vi "6733_88_write_waveform_2014.11.21.vi"(8 "Error In":errorcluster, 9 "Control Reference \nCluster Input":T1, 11 "Red MOT 88 Inputs":T2={"Active Device"="6733_Red_88", "Active Channels"=[TRUE, FALSE, FALSE, FALSE, FALSE, FALSE, FALSE, FALSE], "Waveform Parameters"=[[{"Function"=enum."Polynomial", "Initial"=0.0, "Final"=1.0, "Degree"=1.0, "Nickname"="", "Conversion"=enum."B Field Grad (G/cm)", "Constant"=0.0}, {"Function"=enum."Exponential", "Initial"=0.0, "Final"=0.0, "Degree"=1.0, "Nickname"="", "Conversion"=enum."B Field Grad (G/cm)", "Constant"=0.0}, {"Function"=enum."Exponential", "Initial"=0.0, "Final"=0.0, "Degree"=1.0, "Nickname"="", "Conversion"=enum."B Field Grad (G/cm)", "Constant"=0.0}, {"Function"=enum."Exponential", "Initial"=0.0, "Final"=0.0, "Degree"=1.0, "Nickname"="", "Conversion"=enum."B Field Grad (G/cm)", "Constant"=0.0}, {"Function"=enum."Exponential", "Initial"=0.0, "Final"=0.0, "Degree"=1.0, "Nickname"="", "Conversion"=enum."B Field Grad (G/cm)", "Constant"=0.0}, {"Function"=enum."Exponential", "Initial"=0.0, "Final"=0.0, "Degree"=1.0, "Nickname"="", "Conversion"=enum."B Field Grad (G/cm)", "Constant"=0.0}], [{"Function"=enum."Exponential", "Initial"=0.0, "Final"=0.0, "Degree"=1.0, "Nickname"="", "Conversion"=enum."B Field Grad (G/cm)", "Constant"=0.0}, {"Function"=enum."Exponential", "Initial"=0.0, "Final"=0.0, "Degree"=1.0, "Nickname"="", "Conversion"=enum."B Field Grad (G/cm)", "Constant"=0.0}, {"Function"=enum."Exponential", "Initial"=0.0, "Final"=0.0, "Degree"=1.0, "Nickname"="", "Conversion"=enum."B Field Grad (G/cm)", "Constant"=0.0}, {"Function"=enum."Exponential", "Initial"=0.0, "Final"=0.0, "Degree"=1.0, "Nickname"="", "Conversion"=enum."B Field Grad (G/cm)", "Constant"=0.0}, {"Function"=enum."Exponential", "Initial"=0.0, "Final"=0.0, "Degree"=1.0, "Nickname"="", "Conversion"=enum."B Field Grad (G/cm)", "Constant"=0.0}, {"Function"=enum."Exponential", "Initial"=0.0, "Final"=0.0, "Degree"=1.0, "Nickname"="", "Conversion"=enum."B Field Grad (G/cm)", "Constant"=0.0}], [{"Function"=enum."Exponential", "Initial"=0.0, "Final"=0.0, "Degree"=1.0, "Nickname"="", "Conversion"=enum."B Field Grad (G/cm)", "Constant"=0.0}, {"Function"=enum."Exponential", "Initial"=0.0, "Final"=0.0, "Degree"=1.0, "Nickname"="", "Conversion"=enum."B Field Grad (G/cm)", "Constant"=0.0}, {"Function"=enum."Exponential", "Initial"=0.0, "Final"=0.0, "Degree"=1.0, "Nickname"="", "Conversion"=enum."B Field Grad (G/cm)", "Constant"=0.0}, {"Function"=enum."Exponential", "Initial"=0.0, "Final"=0.0, "Degree"=1.0, "Nickname"="", "Conversion"=enum."B Field Grad (G/cm)", "Constant"=0.0}, {"Function"=enum."Exponential", "Initial"=0.0, "Final"=0.0, "Degree"=1.0, "Nickname"="", "Conversion"=enum."B Field Grad (G/cm)", "Constant"=0.0}, {"Function"=enum."Exponential", "Initial"=0.0, "Final"=0.0, "Degree"=1.0, "Nickname"="", "Conversion"=enum."B Field Grad (G/cm)", "Constant"=0.0}], [{"Function"=enum."Exponential", "Initial"=0.0, "Final"=0.0, "Degree"=1.0, "Nickname"="", "Conversion"=enum."B Field Grad (G/cm)", "Constant"=0.0}, {"Function"=enum."Exponential", "Initial"=0.0, "Final"=0.0, "Degree"=1.0, "Nickname"="", "Conversion"=enum."B Field Grad (G/cm)", "Constant"=0.0}, {"Function"=enum."Exponential", "Initial"=0.0, "Final"=0.0, "Degree"=1.0, "Nickname"="", "Conversion"=enum."B Field Grad (G/cm)", "Constant"=0.0}, {"Function"=enum."Exponential", "Initial"=0.0, "Final"=0.0, "Degree"=1.0, "Nickname"="", "Conversion"=enum."B Field Grad (G/cm)", "Constant"=0.0}, {"Function"=enum."Exponential", "Initial"=0.0, "Final"=0.0, "Degree"=1.0, "Nickname"="", "Conversion"=enum."B Field Grad (G/cm)", "Constant"=0.0}, {"Function"=enum."Exponential", "Initial"=0.0, "Final"=0.0, "Degree"=1.0, "Nickname"="", "Conversion"=enum."B Field Grad (G/cm)", "Constant"=0.0}], [{"Function"=enum."Exponential", "Initial"=0.0, "Final"=0.0, "Degree"=1.0, "Nickname"="", "Conversion"=enum."B Field Grad (G/cm)", "Constant"=0.0}, {"Function"=enum."Exponential", "Initial"=0.0, "Final"=0.0, "Degree"=1.0, "Nickname"="", "Conversion"=enum."B Field Grad (G/cm)", "Constant"=0.0}, {"Function"=enum."Exponential", "Initial"=0.0, "Final"=0.0, "Degree"=1.0, "Nickname"="", "Conversion"=enum."B Field Grad (G/cm)", "Constant"=0.0}, {"Function"=enum."Exponential", "Initial"=0.0, "Final"=0.0, "Degree"=1.0, "Nickname"="", "Conversion"=enum."B Field Grad (G/cm)", "Constant"=0.0}, {"Function"=enum."Exponential", "Initial"=0.0, "Final"=0.0, "Degree"=1.0, "Nickname"="", "Conversion"=enum."B Field Grad (G/cm)", "Constant"=0.0}, {"Function"=enum."Exponential", "Initial"=0.0, "Final"=0.0, "Degree"=1.0, "Nickname"="", "Conversion"=enum."B Field Grad (G/cm)", "Constant"=0.0}], [{"Function"=enum."Exponential", "Initial"=0.0, "Final"=0.0, "Degree"=1.0, "Nickname"="", "Conversion"=enum."B Field Grad (G/cm)", "Constant"=0.0}, {"Function"=enum."Exponential", "Initial"=0.0, "Final"=0.0, "Degree"=1.0, "Nickname"="", "Conversion"=enum."B Field Grad (G/cm)", "Constant"=0.0}, {"Function"=enum."Exponential", "Initial"=0.0, "Final"=0.0, "Degree"=1.0, "Nickname"="", "Conversion"=enum."B Field Grad (G/cm)", "Constant"=0.0}, {"Function"=enum."Exponential", "Initial"=0.0, "Final"=0.0, "Degree"=1.0, "Nickname"="", "Conversion"=enum."B Field Grad (G/cm)", "Constant"=0.0}, {"Function"=enum."Exponential", "Initial"=0.0, "Final"=0.0, "Degree"=1.0, "Nickname"="", "Conversion"=enum."B Field Grad (G/cm)", "Constant"=0.0}, {"Function"=enum."Exponential", "Initial"=0.0, "Final"=0.0, "Degree"=1.0, "Nickname"="", "Conversion"=enum."B Field Grad (G/cm)", "Constant"=0.0}], [{"Function"=enum."Exponential", "Initial"=0.0, "Final"=0.0, "Degree"=1.0, "Nickname"="", "Conversion"=enum."B Field Grad (G/cm)", "Constant"=0.0}, {"Function"=enum."Exponential", "Initial"=0.0, "Final"=0.0, "Degree"=1.0, "Nickname"="", "Conversion"=enum."B Field Grad (G/cm)", "Constant"=0.0}, {"Function"=enum."Exponential", "Initial"=0.0, "Final"=0.0, "Degree"=1.0, "Nickname"="", "Conversion"=enum."B Field Grad (G/cm)", "Constant"=0.0}, {"Function"=enum."Exponential", "Initial"=0.0, "Final"=0.0, "Degree"=1.0, "Nickname"="", "Conversion"=enum."B Field Grad (G/cm)", "Constant"=0.0}, {"Function"=enum."Exponential", "Initial"=0.0, "Final"=0.0, "Degree"=1.0, "Nickname"="", "Conversion"=enum."B Field Grad (G/cm)", "Constant"=0.0}, {"Function"=enum."Exponential", "Initial"=0.0, "Final"=0.0, "Degree"=1.0, "Nickname"="", "Conversion"=enum."B Field Grad (G/cm)", "Constant"=0.0}], [{"Function"=enum."Exponential", "Initial"=0.0, "Final"=0.0, "Degree"=1.0, "Nickname"="", "Conversion"=enum."B Field Grad (G/cm)", "Constant"=0.0}, {"Function"=enum."Exponential", "Initial"=0.0, "Final"=0.0, "Degree"=1.0, "Nickname"="", "Conversion"=enum."B Field Grad (G/cm)", "Constant"=0.0}, {"Function"=enum."Exponential", "Initial"=0.0, "Final"=0.0, "Degree"=1.0, "Nickname"="", "Conversion"=enum."B Field Grad (G/cm)", "Constant"=0.0}, {"Function"=enum."Exponential", "Initial"=0.0, "Final"=0.0, "Degree"=1.0, "Nickname"="", "Conversion"=enum."B Field Grad (G/cm)", "Constant"=0.0}, {"Function"=enum."Exponential", "Initial"=0.0, "Final"=0.0, "Degree"=1.0, "Nickname"="", "Conversion"=enum."B Field Grad (G/cm)", "Constant"=0.0}, {"Function"=enum."Exponential", "Initial"=0.0, "Final"=0.0, "Degree"=1.0, "Nickname"="", "Conversion"=enum."B Field Grad (G/cm)", "Constant"=0.0}]], "Active Phases"=[TRUE, FALSE, FALSE, FALSE, FALSE, FALSE], "Phase Times"=[0.1, 0.1, 0.1], "Trigger Channel"="/6733_Red_88/PFI0"} {"Phase Times" format="%.0p"; "Waveform Parameters"."Degree" min=1.0}) -> (0 "error out":errorcluster={"status"=TRUE, "code"=-89125, "source"="6733_88_write_waveform_2014.11.21.vi<append>\n<B>Source Device: </B>6733_Red_88\n<B>Destination Device: </B>6733_Red_87\n\n<B>Task Name: </B>Red MOT 88 Wfm"}, 2 "counter task out":refnum<k21>, 3 "waveform task out":refnum<k21>="Red MOT 88 Wfm")   [LabVIEW 2016]
uses:
  6733_Red_MOT/6733_control_panel.ctl
  6733_Red_MOT/6733_waveform_parameter_array.ctl
  6733_Red_MOT/6733_waveform_item.ctl
  6733_Red_MOT/Neutral_voltage_conversion_control.ctl
  Controls/6733/Trigger_Channel_Selector.ctl
  Control 1.ctl
  <vilib>/DAQmx/write.llb/DAQmx Write (Analog 1D DBL NChan 1Samp).vi
  <vilib>/DAQmx/write.llb/DAQmx Write (Analog 1D Wfm NChan NSamp).vi
  <vilib>/DAQmx/miscellaneous.llb/DAQmx Fill In Error Info.vi
  <vilib>/Waveform/WDTOps.llb/WDT Append Waveforms DBL.vi
  <vilib>/Waveform/WDTOps.llb/WDT Scale Delta t DBL.vi
  <vilib>/DAQmx/configure/timing.llb/DAQmx Timing (Sample Clock).vi
  <vilib>/DAQmx/create/channels.llb/DAQmx Create Channel (CO-Pulse Generation-Frequency).vi
  <vilib>/DAQmx/configure/timing.llb/DAQmx Timing (Implicit).vi
  <vilib>/DAQmx/configure/trigger.llb/DAQmx Start Trigger (Digital Edge).vi
  <resource>/objmgr/daqmx.rc
panel:
  out "Total Time":dbl=0.1
  out "Sample Rate":dbl=163840.0
  out "Waveforms":waveform(dbl)[](graph)
  out "Max Sample Rate":dbl=1000000.0
  out "# Inactive Channels":i32=7
  out "# Active Channels":i16=1
  out "Inactive Channels":tag[](array[tag])=["6733_Red_87/ao1", "6733_Red_87/ao2", "6733_Red_87/ao3", "6733_Red_87/ao4", "6733_Red_87/ao5", "6733_Red_87/ao6", "6733_Red_87/ao7"]
  out "Active Channels":tag[](array[tag])=["6733_Red_87/ao0"]
  out "Samples Written":dbl=16384.0
  out "Voltage Maximum":dbl=10.0
  out "Voltage Minimum":dbl=-10.0
  out "AO.PhysicalChans":tag[](array[tag])=["6733_Red_87/ao0", "6733_Red_87/ao1", "6733_Red_87/ao2", "6733_Red_87/ao3", "6733_Red_87/ao4", "6733_Red_87/ao5", "6733_Red_87/ao6", "6733_Red_87/ao7"]
  out "Active Device":tag="6733_Red_87"
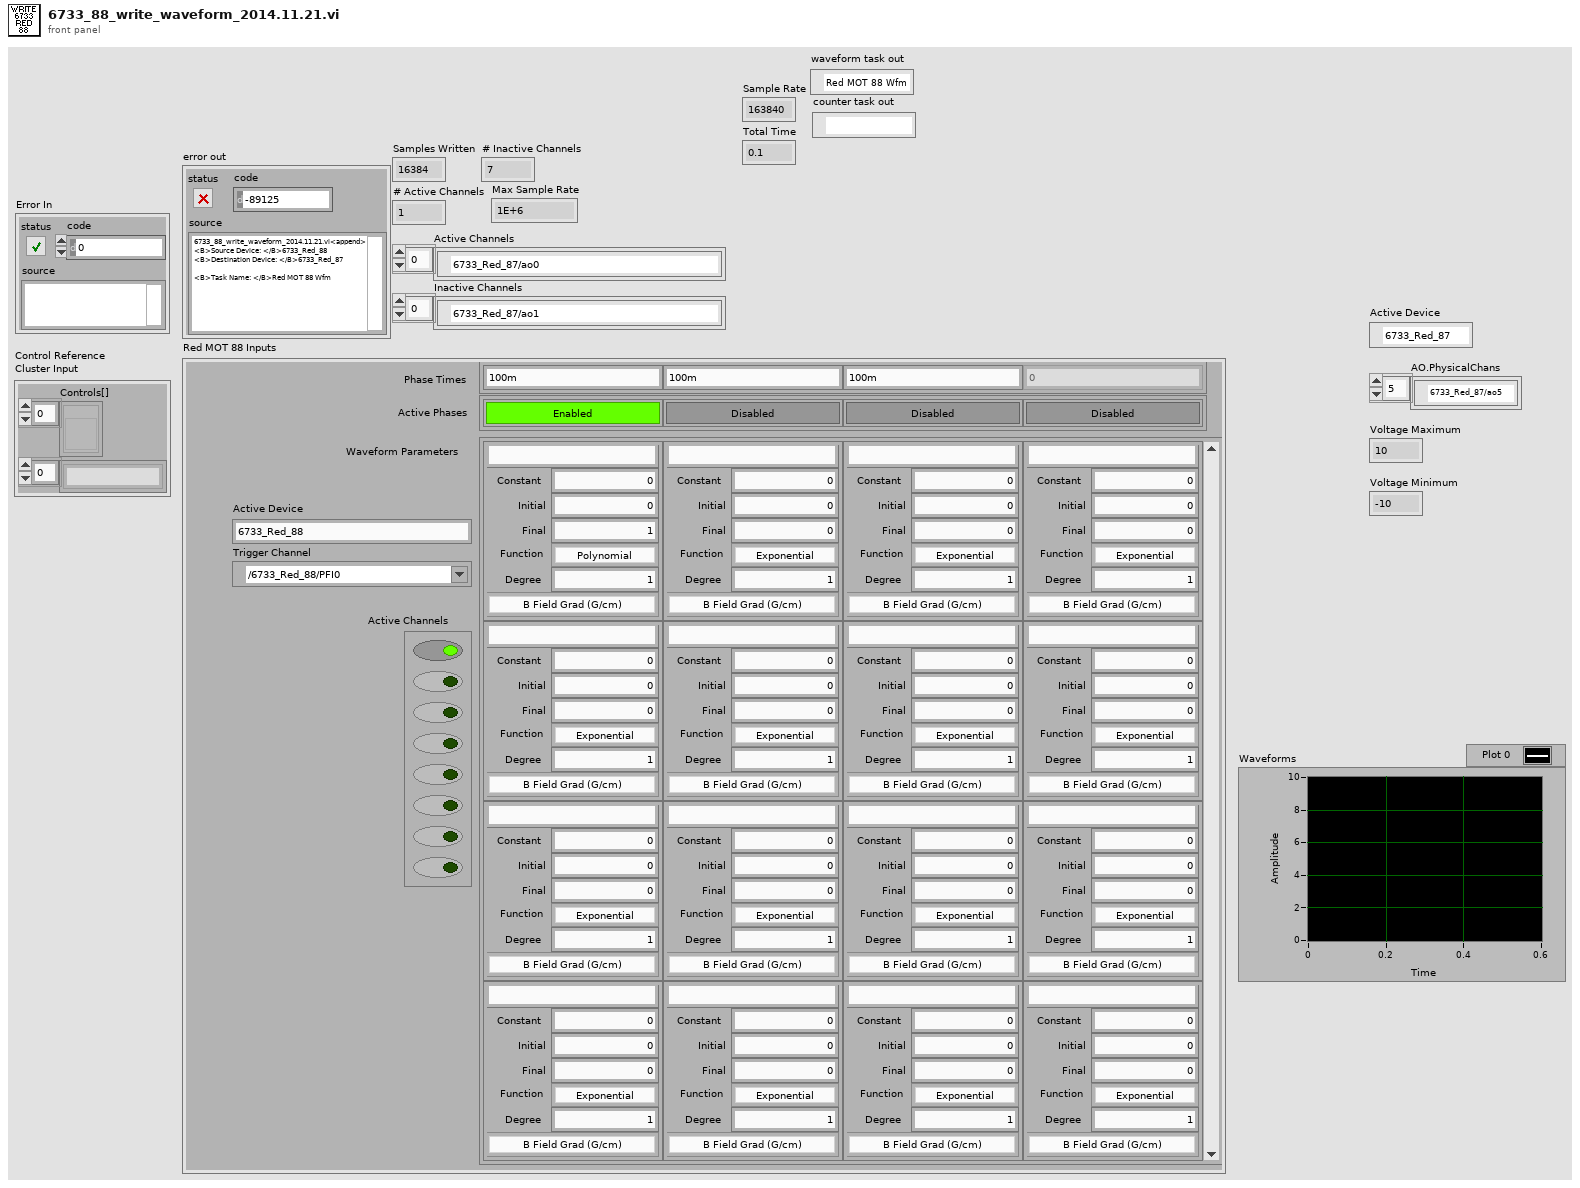
[diagram p1: front panel]
types:
  T1 = cluster{"Controls[]":refnum<vi>[], "Control Names":string[]}
  T2 = typedef "6733_control_panel.ctl" = cluster{"Active Device":string, "Active Channels":bool[], "Waveform Parameters":T3, "Active Phases":bool[], "Phase Times":dbl[], "Trigger Channel":T6}
  T3 = typedef "6733_waveform_parameter_array.ctl" = T4[][]
  T4 = typedef "6733_waveform_item.ctl" = cluster{"Function":enum16{"Polynomial", "Exponential", "Constant", "Tanh"}, "Initial":dbl, "Final":dbl, "Degree":dbl, "Nickname":string, "Conversion":T5, "Constant":dbl}
  T5 = typedef "Neutral_voltage_conversion_control.ctl" = enum16{"Volts", "B Field Grad (G/cm)", "Red Boson Cntr Freq (MHz)", "Red Boson Dither Amp (kHz)", "Red Boson Power (mW)", "Red 87 Trap Cntr Freq (MHz)", "Red 87 Trap Dither Amp (kHz)", "Red 87 Trap Power (mW)", "Red 87 Stir Cntr Freq (MHz)", "Red 87 Stir Dither Amp (kHz)", "Red 87 Stir Power (mW)", "ODT Sheet Trap Power (W)", "ODT Loading Trap Power (W)"}
  T6 = typedef "Trigger_Channel_Selector.ctl" = tag
  T7 = typedef "Control 1.ctl" = enum16{"Initialize", "Get Device Information", "Get Active/Inactive Channels", "Maximize Samples / Channel", "Calculate Waveforms", "Check for Problems", "Update Front Panel", "Clear Old Tasks", "Write Initialization to Cards", "Write Waveform to Cards"}
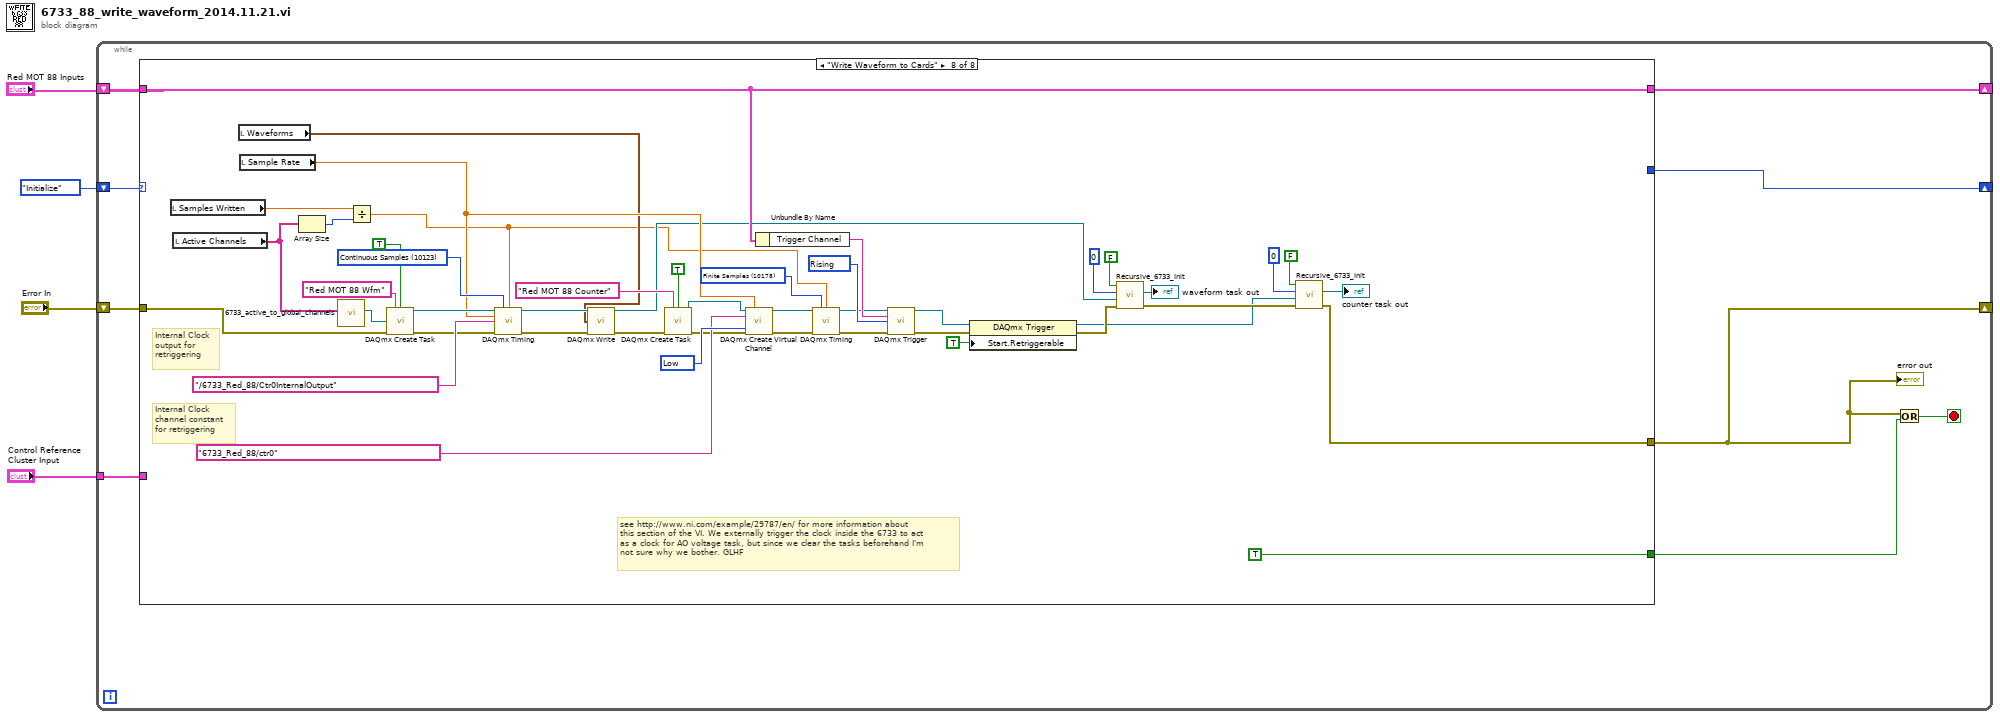
[diagram p0: block diagram]
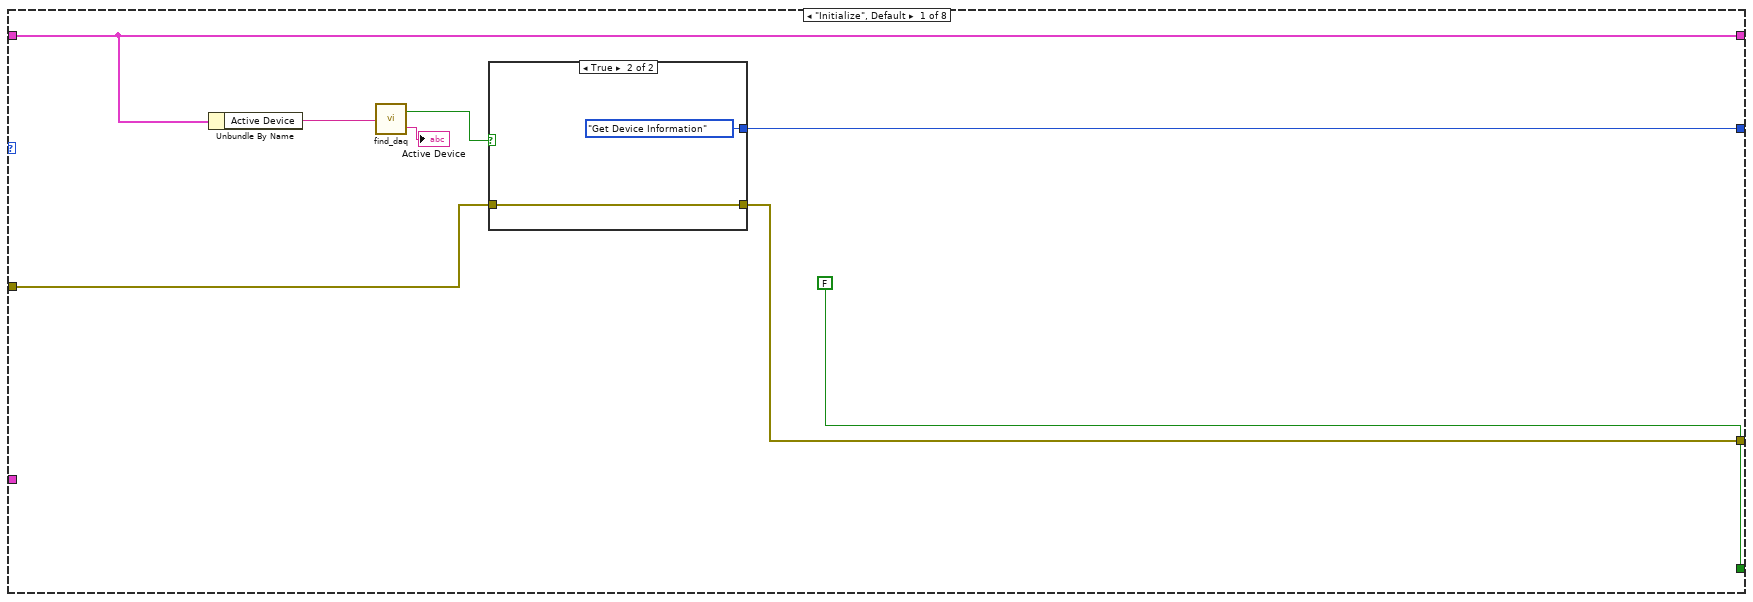
[diagram p2: hidden frame]
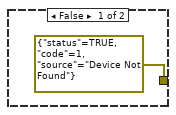
[diagram p3: hidden frame]
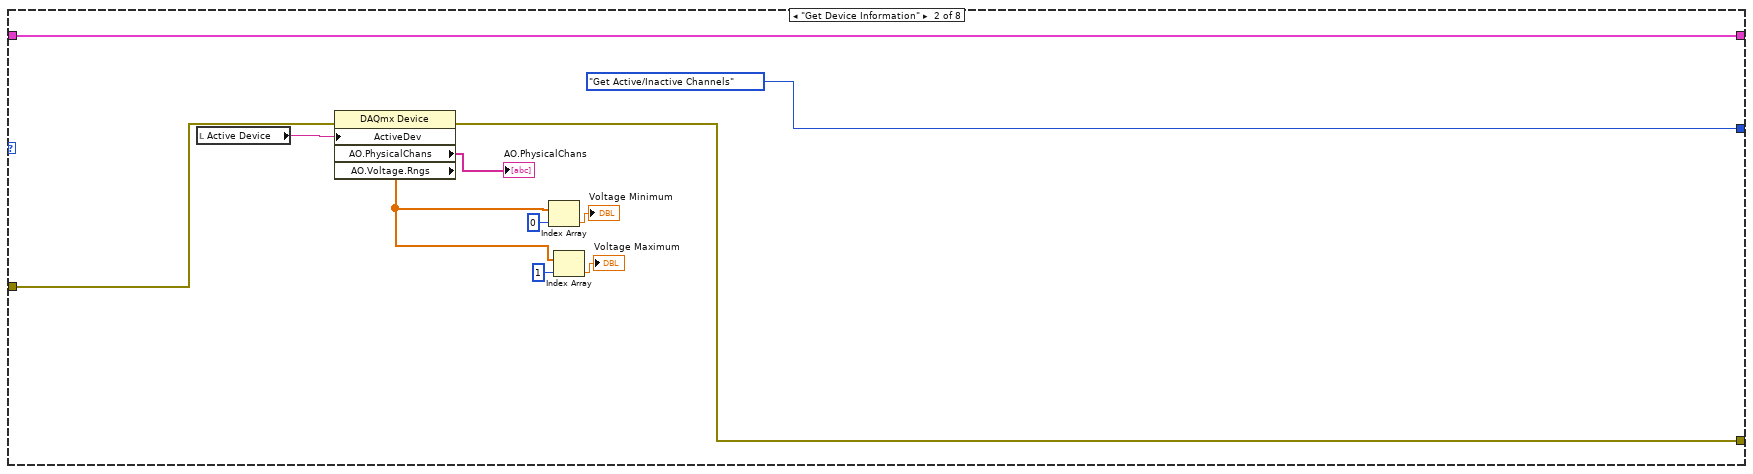
[diagram p4: hidden frame]
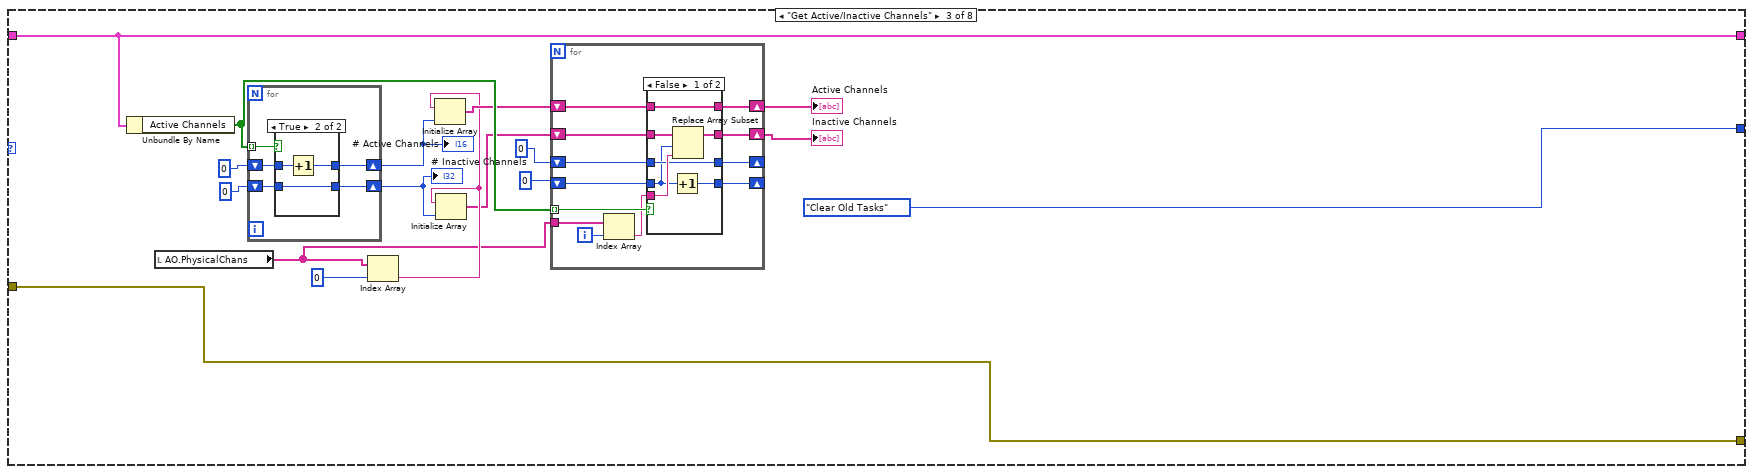
[diagram p5: hidden frame]
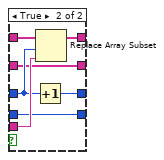
[diagram p6: hidden frame]
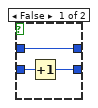
[diagram p7: hidden frame]
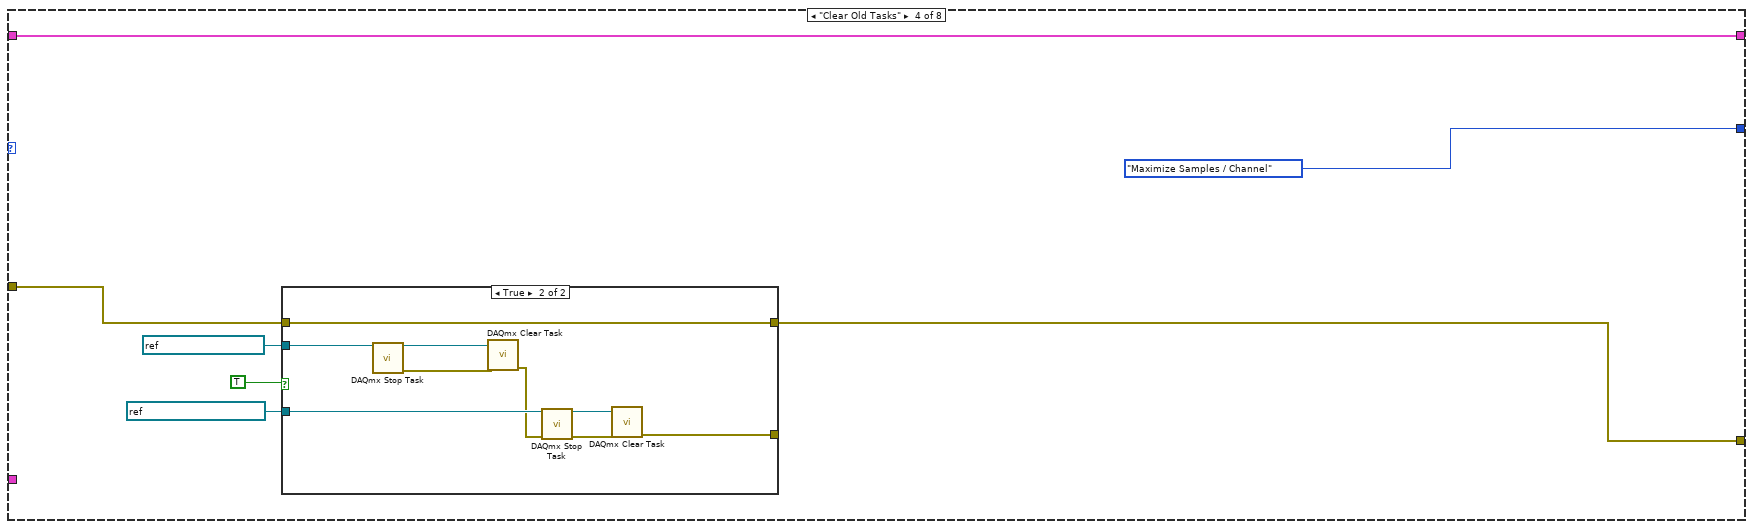
[diagram p8: hidden frame]
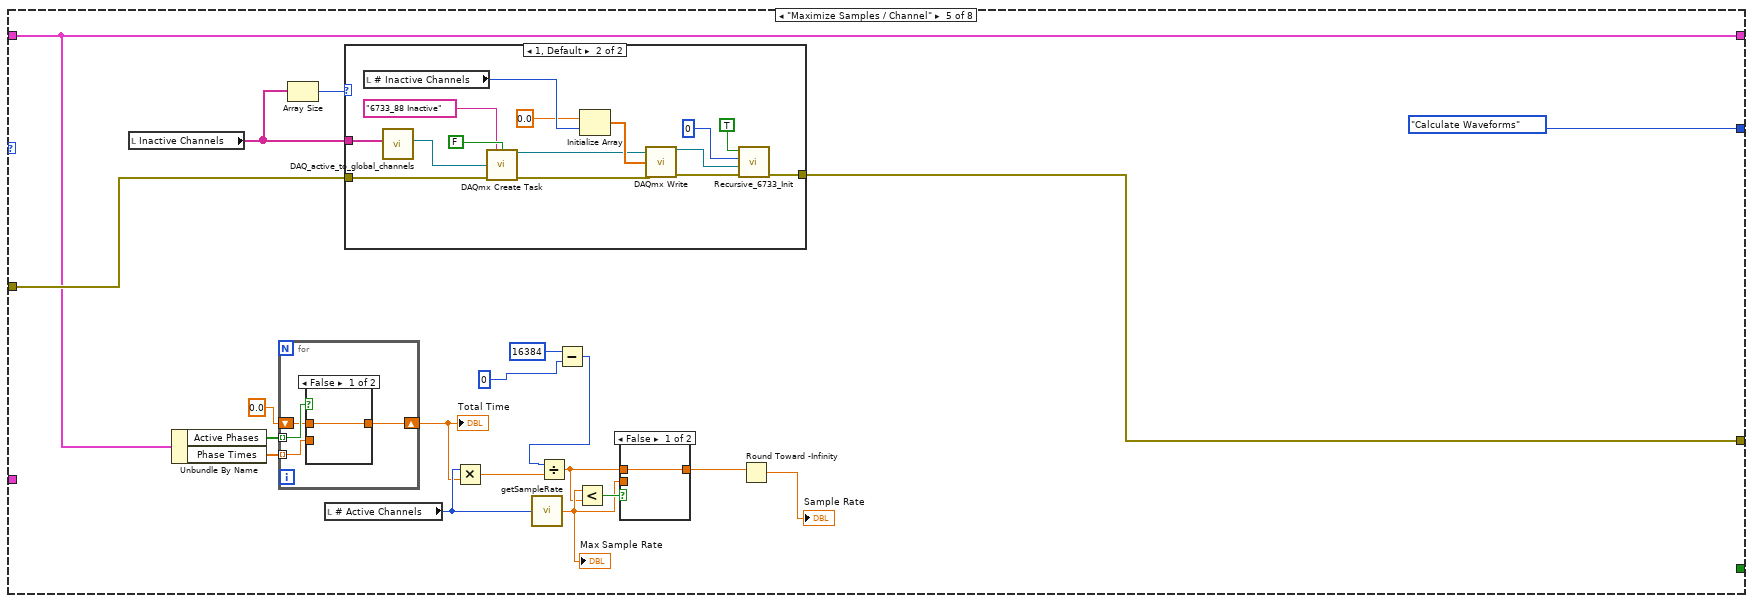
[diagram p10: hidden frame]
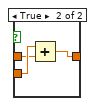
[diagram p13: hidden frame]
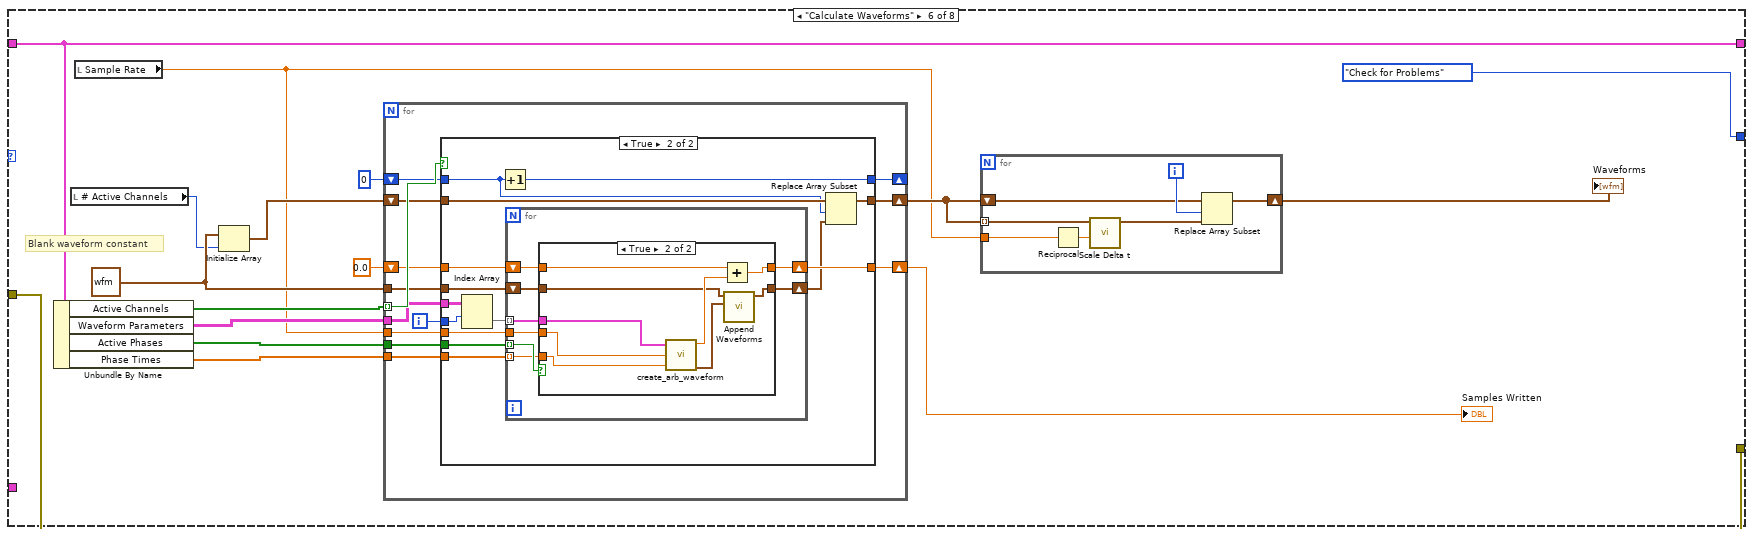
[diagram p14: hidden frame]
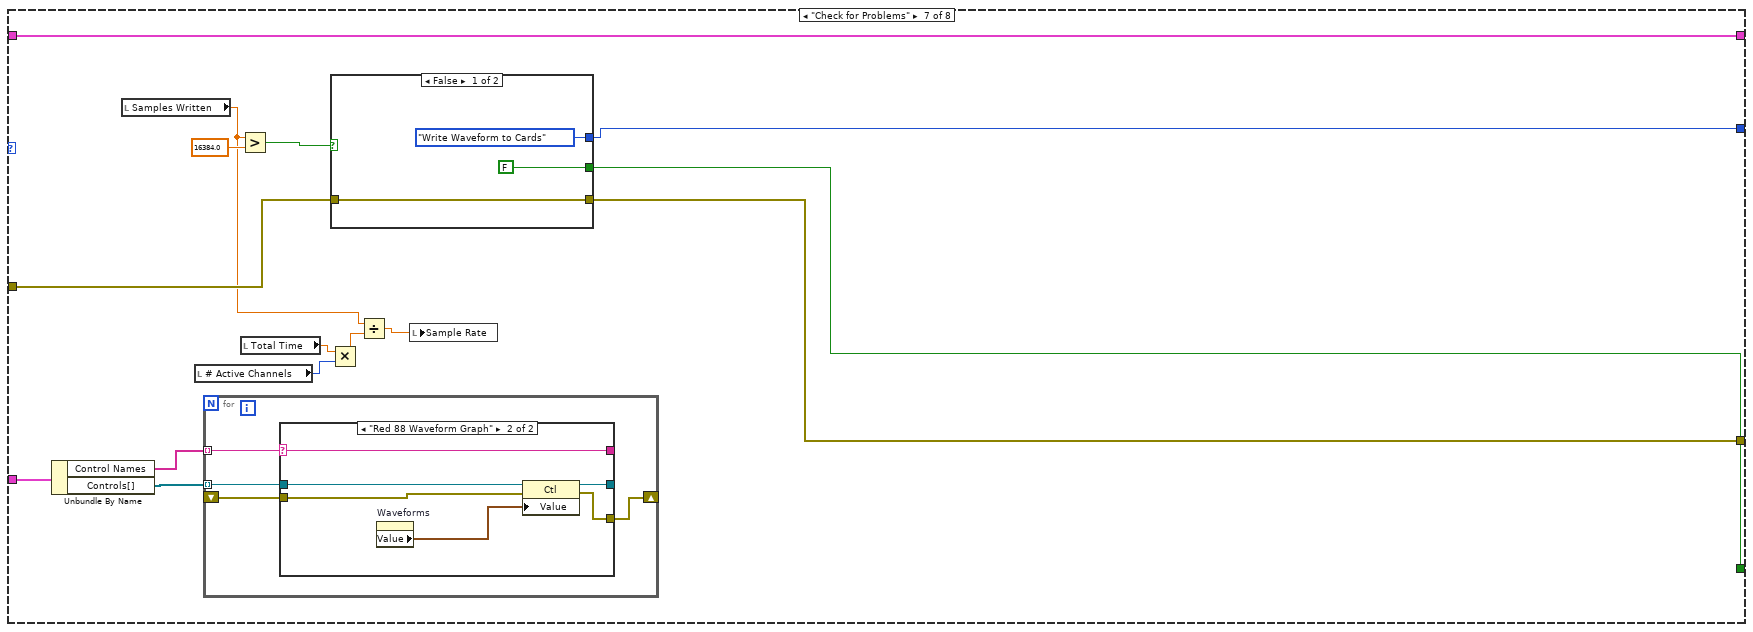
[diagram p17: hidden frame]
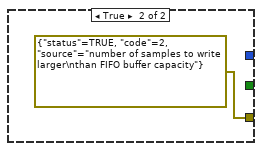
[diagram p19: hidden frame]
diagram:
  n1 = while {
    shift-right: [w9] -> _
    shift-left: "Error In" -> [w11]
    shift-right: [w10] -> _
    shift-left: Control_1."Initialize" -> [w13]
    shift-right: [w7] -> _
    shift-left: "Red MOT 88 Inputs" -> [w12]
    tunnel: "Control Reference \nCluster Input" -> [w5]
    stop <- w8 stop-if-true
    n2 = case shown="\"Write Waveform to Cards\"" w13 {
      tunnel: w12 -> [w15 w35 w39 w92 w123 w164 w228 w301]
      tunnel: [w18 w26 w50 w95 w125 w167 w236 w263] -> w9
      tunnel: w11 -> [w17 w34 w50 w94 w126 w167 w237 w284]
      tunnel: [w16 Control_1."Get Active/Inactive Channels" Control_1."Clear Old Tasks" Control_1."Maximize Samples / Channel" Control_1."Calculate Waveforms" Control_1."Check for Problems" w235 _] -> w10
      tunnel: [w15 w35 w39 w92 w123 w164 w228 w301] -> w7
      tunnel: [FALSE ("y") _ _ _ _ _ w234 TRUE ("y")] -> w6
      tunnel: w5 -> [_ _ _ _ _ _ w225 _]
      frame "Initialize", Default {
        n3 = Unbundle By Name(w15) -> ("Active Device"=w21:string)
        n4 = call "find_daq.vi"("Device Name"=w21) -> ("Device Present"=w19:bool, "DAQmx Device Name"=→"Active Device":tag)
        n5 = case shown="True" w19 {
          tunnel: [errorcluster {"status"=TRUE, "code"=1, "source"="Device Not Found"} ("error in (no error)") w24] -> w18
          tunnel: w17 -> [_ w24]
          tunnel: [_ Control_1."Get Device Information"] -> w16
          frame False {
          }
          frame True {
          }
        }
      }
      frame "Get Device Information" {
        n6 = local read "Active Device"() -> (w33:tag)
        n7 = property class="DAQmx Device"(error in=w34, "ActiveDev"=w33) -> (error out=w26:errorcluster, "AO.PhysicalChans"=→"AO.PhysicalChans":tag[], "AO.Voltage.Rngs"=w28:dbl[])  [unwired: 1 in, 1 out]
        n8 = Index Array(array=w28, index=0) -> (element=→"Voltage Minimum":dbl)
        n9 = Index Array(array=w28, index=1) -> (element=→"Voltage Maximum":dbl)
      }
      frame "Get Active/Inactive Channels" {
        n10 = Unbundle By Name(w39) -> ("Active Channels"=w49:bool[])
        n11 = local read "AO.PhysicalChans"() -> (w43:tag[])
        n12 = for {
          shift-right: [w83] -> w48
          shift-left: i16 0 -> [w82]
          shift-right: [w81] -> w47
          shift-left: 0 -> [w80]
          tunnel: w49 -> [w79] mode=indexing
          n13 = case shown="True" w79 {
            tunnel: [w84 w89] -> w83
            tunnel: w82 -> [w84 w88]
            tunnel: [w86 w87] -> w81
            tunnel: w80 -> [w85 w87]
            frame False {
              n14 = Increment(x=w85) -> (x+1=w86:i32)
            }
            frame True {
              n15 = Increment(x=w88) -> (x+1=w89:i16)
            }
          }
        }
        "# Active Channels" <- w48
        "# Inactive Channels" <- w47
        n16 = Index Array(array=w43, index=0) -> (element=w44:tag)
        n17 = Initialize Array(w44, w48) -> (w46:tag[])
        n18 = Initialize Array(w44, w47) -> (w42:tag[])
        n19 = for {
          tunnel: w49 -> [w64] mode=indexing
          shift-right: [w61] -> w38
          shift-left: w46 -> [w62]
          tunnel: w43 -> [w59]
          shift-right: [w57] -> w37
          shift-left: w42 -> [w58]
          shift-right: [w55] -> _
          shift-left: 0 ("index") -> [w56]
          shift-right: [w53] -> _
          shift-left: 0 ("index") -> [w54]
          i -> [w63]
          n20 = Index Array(array=w59, index=w63) -> (element=w60:tag)
          n21 = case shown="False" w64 {
            tunnel: w62 -> [w65 w78]
            tunnel: [w65 w77] -> w61
            tunnel: w60 -> [w71 w76]
            tunnel: w58 -> [w70 w72]
            tunnel: [w69 w72] -> w57
            tunnel: w56 -> [w68 w75]
            tunnel: [w68 w74] -> w55
            tunnel: w54 -> [w67 w73]
            tunnel: [w66 w73] -> w53
            frame False {
              n22 = Increment(x=w67) -> (x+1=w66:i32)
              n23 = Replace Array Subset(array=w70, new element=w71, index=w67) -> (w69:tag[])
            }
            frame True {
              n24 = Increment(x=w75) -> (x+1=w74:i32)
              n25 = Replace Array Subset(array=w78, new element=w76, index=w75) -> (w77:tag[])
            }
          }
        }
        "Active Channels" <- w38
        "Inactive Channels" <- w37
      }
      frame "Clear Old Tasks" {
        n26 = case shown="True" TRUE {
          tunnel: refnum<k21> "Red MOT 88 Wfm" ("Waveform Task In") -> [_ w106]
          tunnel: refnum<k21> "Red MOT 88 Counter" ("Control Task In") -> [_ w104]
          tunnel: [w97 w102] -> w95
          tunnel: w94 -> [w97 w102]
          tunnel: [_ w98] -> _
          frame False {
          }
          frame True {
            n27 = call <vilib>:"DAQmx Stop Task.vi"("task/channels in"=w106) -> ("task out"=w105:refnum<k21>, "error out"=w101:errorcluster)  [unwired: 13 in]
            n28 = call <vilib>:"DAQmx Clear Task.vi"("task in"=w105, "error in"=w101) -> ("error out"=w100:errorcluster)  [unwired: 13 in]
            n29 = call <vilib>:"DAQmx Stop Task.vi"("task/channels in"=w104, "error in"=w100) -> ("task out"=w103:refnum<k21>, "error out"=w99:errorcluster)  [unwired: 12 in]
            n30 = call <vilib>:"DAQmx Clear Task.vi"("task in"=w103, "error in"=w99) -> ("error out"=w98:errorcluster)  [unwired: 13 in]
          }
        }
      }
      frame "Maximize Samples / Channel" {
        n31 = local read "Inactive Channels"() -> (w108:tag[])
        n32 = Unbundle By Name(w123) -> ("Active Phases"=w122:bool[], "Phase Times"=w121:dbl[])
        n33 = for {
          tunnel: w122 -> [w148] mode=indexing
          tunnel: w121 -> [w147] mode=indexing
          shift-right: [w145] -> w114
          shift-left: 0.0 -> [w146]
          n34 = case shown="False" w148 {
            tunnel: w147 -> [_ w152]
            tunnel: w146 -> [w149 w151]
            tunnel: [w149 w150] -> w145
            frame False {
            }
            frame True {
              n35 = Add(x=w152, y=w151) -> (x+y=w150:dbl)
            }
          }
        }
        "Total Time" <- w114
        n36 = Array Size(array=w108) -> (size(s)=w107:i32)
        n37 = local read "# Active Channels"() -> (w115:i16)
        n38 = case shown="1, Default" w107 {
          tunnel: w126 -> [w127 w134]
          tunnel: [w127 w138] -> w125
          tunnel: w108 -> [_ w135]
          frame 0 {
          }
          frame 1, Default {
            n39 = local read "# Inactive Channels"() -> (w142:i32)
            n40 = call "DAQ_active_to_global_channels.vi"("Active Channels"=w135) -> ("Global Channels"=w136:refnum<k21>)  [unwired: 10 in]
            n41 = call <vilib>:"DAQmx Create Task.vi"("new task name"="6733_88 Inactive", "auto cleanup"=FALSE, "global virtual channels"=w136, "error in"=w134) -> ("task out"=w131:refnum<k21>, "error out"=w132:errorcluster)  [unwired: 10 in]
            n42 = Initialize Array(0.0 ("element"), w142) -> (w140:dbl[])
            n43 = call-poly <vilib>:"DAQmx Write.vi"("task/channels in"=w131, "data"=w140, "error in"=w132) -> ("task out"=w130:refnum<k21>, "error out"=w139:errorcluster)  [unwired: 10 in, 1 out]
            n44 = call "Recursive_6733_Init.vi"("Error In"=w139, "task in"=w130, "Counter"=0, "Stop and Clear?"=TRUE) -> ("error out"=w138:errorcluster)  [unwired: 2 in, 1 out]
          }
        }
        n45 = Multiply(x=w115, y=w114) -> (x*y=w116:dbl)
        n46 = call "getSampleRate.vi"("Number of active channels"=w115) -> ("Sample Rate"=w118:dbl)
        "Max Sample Rate" <- w118
        n47 = Subtract(x=16384, y=0) -> (x-y=w112:i32)
        n48 = Divide(x=w112, y=w116) -> (x/y=w117:dbl)
        n49 = Less?(x=w118, y=w117) -> (x < y?=w119:bool)
        n50 = case shown="False" w119 {
          tunnel: [w143 w144] -> w110
          tunnel: w118 -> [_ w144]
          tunnel: w117 -> [w143 _]
          frame False {
          }
          frame True {
          }
        }
        n51 = Round Toward -Infinity(1:w110) -> (0:→"Sample Rate":dbl)
      }
      frame "Calculate Waveforms" {
        w161 = waveform(dbl) {"t0"=timestamp(0 s since 1904-01-01), "dt"=1.0, "Y"=[]}
        # "Blank waveform constant"
        n52 = Unbundle By Name(w164) -> ("Active Channels"=w157:bool[], "Waveform Parameters"=w168:T3, "Active Phases"=w162:bool[], "Phase Times"=w158:dbl[])
        n53 = local read "# Active Channels"() -> (w156:i16)
        n54 = local read "Sample Rate"() -> (w153:dbl)
        n55 = Initialize Array(w161, w156) -> (w159:waveform(dbl)[])
        n56 = for {
          tunnel: w157 -> [w188] mode=indexing
          tunnel: w168 -> [w186]
          shift-right: [w185] -> w166
          shift-left: 0.0 -> [w184]
          tunnel: w162 -> [w183]
          tunnel: w161 -> [w182]
          shift-right: [w180] -> _
          shift-left: 0 -> [w181]
          shift-right: [w178] -> w155
          shift-left: w159 -> [w179]
          tunnel: w158 -> [w177]
          tunnel: w153 -> [w176]
          i -> [w187]
          n57 = case shown="True" w188 {
            tunnel: w187 -> [_ w205]
            tunnel: w186 -> [_ w204]
            tunnel: [w191 w203] -> w185
            tunnel: w184 -> [w191 w202]
            tunnel: w183 -> [_ w200]
            tunnel: w182 -> [_ w199]
            tunnel: w181 -> [w190 w196]
            tunnel: [w190 w198] -> w180
            tunnel: w179 -> [w189 w197]
            tunnel: [w189 w194] -> w178
            tunnel: w177 -> [_ w193]
            tunnel: w176 -> [_ w192]
            frame False {
            }
            frame True {
              n58 = Index Array(array=w204, index (row)=w205) -> (element=w201:T4[])  [unwired: 1 in]
              n59 = Increment(x=w196) -> (x+1=w198:i32)
              n60 = for {
                shift-right: [w213] -> w203
                shift-left: w202 -> [w212]
                tunnel: w201 -> [w211] mode=indexing
                shift-right: [w209] -> w195
                shift-left: w199 -> [w210]
                tunnel: w200 -> [w208] mode=indexing
                tunnel: w193 -> [w207] mode=indexing
                tunnel: w192 -> [w206]
                n61 = case shown="True" w208 {
                  tunnel: [w215 w223] -> w213
                  tunnel: w212 -> [w215 w222]
                  tunnel: w211 -> [_ w218]
                  tunnel: w210 -> [w214 w220]
                  tunnel: [w214 w219] -> w209
                  tunnel: w207 -> [_ w217]
                  tunnel: w206 -> [_ w216]
                  frame False {
                  }
                  frame True {
                    n62 = call "create_arb_waveform.vi"("Waveform Parameters"=w218, "Sample rate"=w216, "Time"=w217) -> ("Samples to Write"=w224:dbl, "output waveform"=w221:waveform(dbl))  [unwired: 2 out]
                    n63 = Add(x=w222, y=w224) -> (x+y=w223:dbl)
                    n64 = call-poly <vilib>:"Append Waveforms.vi"("waveform B"=w221, "waveform A"=w220) -> ("waveform out"=w219:waveform(dbl))  [unwired: 8 in, 1 out]
                  }
                }
              }
              n65 = Replace Array Subset(array=w197, new element=w195, index=w196) -> (w194:waveform(dbl)[])
            }
          }
        }
        "Samples Written" <- w166
        n66 = for {
          tunnel: w155 -> [w175] mode=indexing
          shift-right: [w169] -> w154
          shift-left: w155 -> [w171]
          tunnel: w153 -> [w170]
          i -> [w173]
          n67 = Reciprocal(x=w170) -> (1/x=w174:dbl)
          n68 = call-poly <vilib>:"Scale Delta t.vi"("scale factor"=w174, "waveform in"=w175) -> ("waveform out"=w172:waveform(dbl))  [unwired: 8 in, 1 out]
          n69 = Replace Array Subset(array=w171, new element=w172, index=w173) -> (w169:waveform(dbl)[])
        }
        "Waveforms" <- w154
      }
      frame "Check for Problems" {
        n70 = Unbundle By Name(w225) -> ("Control Names"=w227:string[], "Controls[]"=w226:refnum<vi>[])
        n71 = local read "Samples Written"() -> (w233:dbl)
        n72 = local read "# Active Channels"() -> (w230:i16)
        n73 = for {
          tunnel: w227 -> [w243] mode=indexing
          shift-right: [w240] -> _
          shift-left: _ -> [w241]
          tunnel: w226 -> [w242] mode=indexing
          n74 = case shown="\"Red 88 Waveform Graph\"" w243 {
            selector: w243 -> [w246 w252]
            tunnel: w242 -> [w245 w249]
            tunnel: [w246 w252] -> _
            tunnel: [w245 w248] -> _
            tunnel: w241 -> [w244 w251]
            tunnel: [w244 w250] -> w240
            frame "False", Default {
            }
            frame "Red 88 Waveform Graph" {
              n75 = property on="Waveforms" class="WFGraph (strict)"() -> ("Value"=w247:waveform(dbl)[])  [unwired: 2 in, 2 out]
              n76 = property class="Ctl"(reference=w249, error in=w251, "Value"=w247) -> (reference out=w248:refnum<vi>, error out=w250:errorcluster)
            }
          }
        }
        n77 = Greater?(x=w233, y=16384.0) -> (0:w239:bool)
        n78 = local read "Total Time"() -> (w231:dbl)
        n79 = Multiply(x=w231, y=w230) -> (x*y=w229:dbl)
        n80 = case shown="False" w239 {
          tunnel: w237 -> [w255 _]
          tunnel: [w255 errorcluster {"status"=TRUE, "code"=2, "source"="number of samples to write larger\nthan FIFO buffer capacity"} ("error in (no error)")] -> w236
          tunnel: [Control_1."Write Waveform to Cards" _] -> w235
          tunnel: [FALSE ("y") _] -> w234
          frame False {
          }
          frame True {
          }
        }
        n81 = Divide(x=w233, y=w229) -> (x/y=w232:dbl)
        n82 = local write "Sample Rate"(w232) -> ()
      }
      frame "Write Waveform to Cards" {
        w292 = 10280 items=["Rising"=10280, "Falling"=10171] ("edge")
        w296 = 10123 items=["Finite Samples"=10178, "Continuous Samples"=10123, "Hardware Timed Single Point"=12522] ("sample mode")
        w297 = 10178 items=["Finite Samples"=10178, "Continuous Samples"=10123, "Hardware Timed Single Point"=12522] ("sample mode")
        w300 = 10214 items=["High"=10192, "Low"=10214] ("idle state")
        # "see http://www.ni.com/example/29787/en/ for more information about\nthis section of the VI. We externally trigger the clock inside the 6733 to act\nas a clock for AO voltage task, but since we clear the tasks beforehand I'm\nnot sure why we bother. GLHF"
        # "Internal Clock\noutput for\nretriggering"
        # "Internal Clock\nchannel constant\nfor retriggering"
        n83 = local read "Samples Written"() -> (w257:dbl)
        n84 = local read "Active Channels"() -> (w258:tag[])
        n85 = local read "Waveforms"() -> (w272:waveform(dbl)[])
        n86 = local read "Sample Rate"() -> (w273:dbl)
        n87 = Array Size(array=w258) -> (size(s)=w259:i32)
        n88 = call "6733_active_to_global_channels.vi"("Active Channels"=w258) -> ("Global Channels"=w282:refnum<k21>)  [unwired: 10 in]
        n89 = Divide(x=w257, y=w259) -> (x/y=w260:dbl)
        n90 = call <vilib>:"DAQmx Create Task.vi"("new task name"="Red MOT 88 Wfm", "auto cleanup"=TRUE, "global virtual channels"=w282, "error in"=w284) -> ("task out"=w280:refnum<k21>, "error out"=w283:errorcluster)  [unwired: 10 in]
        n91 = call-poly <vilib>:"DAQmx Timing.vi"("task/channels in"=w280, "sample mode"=w296, "samples per channel"=w260, "rate"=w273, "source"=tag "/6733_Red_88/Ctr0InternalOutput", "error in"=w283) -> ("task out"=w294:refnum<k21>, "error out"=w295:errorcluster)  [unwired: 8 in]
        n92 = call-poly <vilib>:"DAQmx Write.vi"("task/channels in"=w294, "data"=w272, "error in"=w295) -> ("task out"=w270:refnum<k21>, "error out"=w279:errorcluster)  [unwired: 10 in, 1 out]
        n93 = call <vilib>:"DAQmx Create Task.vi"("new task name"="Red MOT 88 Counter", "auto cleanup"=TRUE, "error in"=w279) -> ("task out"=w274:refnum<k21>, "error out"=w278:errorcluster)  [unwired: 11 in]
        n94 = call-poly <vilib>:"DAQmx Create Virtual Channel.vi"("task in"=w274, "frequency"=w273, "counter"=tag "6733_Red_88/ctr0", "error in"=w278, "idle state"=w300) -> ("task out"=w299:refnum<k21>, "error out"=w298:errorcluster)  [unwired: 9 in]
        n95 = Unbundle By Name(w301) -> ("Trigger Channel"=w291:T6)
        n96 = call-poly <vilib>:"DAQmx Timing.vi"("task/channels in"=w299, "sample mode"=w297, "samples per channel"=w260, "error in"=w298) -> ("task out"=w290:refnum<k21>, "error out"=w293:errorcluster)  [unwired: 10 in]
        n97 = call-poly <vilib>:"DAQmx Trigger.vi"("task/channels in"=w290, "source"=w291, "edge"=w292, "error in"=w293) -> ("task out"=w288:refnum<k21>, "error out"=w289:errorcluster)  [unwired: 10 in]
        n98 = property class="DAQmx Trigger"(reference=w288, error in=w289, "Start.Retriggerable"=TRUE) -> (reference out=w262:refnum<k21>, error out=w271:errorcluster)
        n99 = call "Recursive_6733_Init.vi"("Error In"=w271, "task in"=w270, "Counter"=0, "Stop and Clear?"=FALSE) -> ("error out"=w264:errorcluster, "task out"=→"waveform task out":refnum<k21>)  [unwired: 2 in]
        n100 = call "Recursive_6733_Init.vi"("Error In"=w264, "task in"=w262, "Counter"=0, "Stop and Clear?"=FALSE) -> ("error out"=w263:errorcluster, "task out"=→"counter task out":refnum<k21>)  [unwired: 2 in]
      }
    }
    "error out" <- w9
    n101 = Or(x=w9, y=w6) -> (x .or. y?=w8:bool)
  }
